vi "CRYCal Perceptual Rub&buzz HarmonicTrack.vi"(6 "Fs":dbl=44100.0, 8 "TSR params":T2={"FSamp"=44100.0, "FStart"=20.0, "FStop"=20000.0, "NOffset"=0.0, "MStop"=132741.0, "MStart"=441.0, "NHarm"=19152.386651933408, "Tsamp"=2.2675736961451248e-05, "Amplit"=1.0, "Sweep Time"=1.0} {"Sweep Time" format="%.2f"; "Amplit" format="%.2f"; "FStop" format="%.2f"; "FStart" format="%.2f"; "FSamp" format="%.2f"; "Tsamp" format="%.2f"; "NHarm" format="%.2f"; "MStart" format="%.2f"; "MStop" format="%.2f"; "NOffset" format="%.2f"}, 9 "Harmonic Infor":T1={"Cycles"=[200.0, 190.0, 180.0, 170.0, 160.0, 150.0, 140.0, 132.0, 125.0, 118.0, 112.0, 106.0, 100.0, 95.0, 90.0, 85.0, 80.0, 75.0, 71.0, 67.0, 63.0, 60.0, 56.0, 53.0, 50.0, 48.0, 45.0, 43.0, 40.0, 38.0, 36.0, 34.0, 32.0, 30.0, 28.0, 27.0, 25.0, 24.0, 23.0, 22.0, 20.0, 19.0, 18.0, 17.0, 16.0, 15.0, 14.0, 14.0, 13.0, 12.0, 12.0, 11.0, 10.0, 10.0, 9.0, 9.0, 8.0, 8.0, 8.0, 7.0, 7.0, 6.0, 6.0, 6.0, 6.0, 6.0, 6.0, 6.0, 6.0, 6.0, 6.0, 6.0, 6.0, 6.0, 8.0, 8.0, 8.0, 8.0, 8.0, 8.0, 8.0, 8.0], "Frequency"=[20000.0, 19000.0, 18000.0, 17000.0, 16000.0, 15000.0, 14000.0, 13199.999809265137, 12500.0, 11800.000190734863, 11199.999809265137, 10600.000381469727, 10000.0, 9500.0, 9000.0, 8500.0, 8000.0, 7500.0, 7099.999904632568, 6699.999809265137, 6300.000190734863, 6000.0, 5599.999904632568, 5300.000190734863, 5000.0, 4750.0, 4500.0, 4250.0, 4000.0, 3750.0, 3549.999952316284, 3349.9999046325684, 3150.0000953674316, 3000.0, 2799.999952316284, 2650.0000953674316, 2500.0, 2359.999895095825, 2240.000009536743, 2119.999885559082, 2000.0, 1900.0, 1800.0, 1700.0, 1600.0, 1500.0, 1400.0, 1319.9999809265137, 1250.0, 1180.0000190734863, 1119.9999809265137, 1060.0000381469727, 1000.0, 950.0, 900.0, 850.0, 800.0, 750.0, 709.9999904632568, 669.9999809265137, 630.0000190734863, 600.0, 559.9999904632568, 530.0000190734863, 500.0, 475.0, 450.0, 425.0, 400.0, 375.0, 354.9999952316284, 334.99999046325684, 315.00000953674316, 300.0, 250.0, 200.0, 160.0, 125.0, 100.0, 80.0, 63.00000190734863, 50.0], "Amplitude"=[0.5, 0.5, 0.5, 0.5, 0.5, 0.5, 0.5, 0.5, 0.5, 0.5, 0.5, 0.5, 0.5, 0.5, 0.5, 0.5, 0.5, 0.5, 0.5, 0.5, 0.5, 0.5, 0.5, 0.5, 0.5, 0.5, 0.5, 0.5, 0.5, 0.5, 0.5, 0.5, 0.5, 0.5, 0.5, 0.5, 0.5, 0.5, 0.5, 0.5, 0.5, 0.5, 0.5, 0.5, 0.5, 0.5, 0.5, 0.5, 0.5, 0.5, 0.5, 0.5, 0.5, 0.5, 0.5, 0.5, 0.5, 0.5, 0.5, 0.5, 0.5, 0.5, 0.5, 0.5, 0.5, 0.5, 0.5, 0.5, 0.5, 0.5, 0.5, 0.5, 0.5, 0.5, 0.5, 0.5, 0.5, 0.5, 0.5, 0.5, 0.5, 0.5], "samples"=[441, 441, 441, 441, 441, 441, 441, 441, 441, 441, 441, 441, 441, 441, 441, 441, 441, 441, 441, 441, 441, 441, 441, 441, 441, 446, 441, 446, 441, 447, 447, 447, 448, 441, 441, 450, 441, 448, 453, 458, 441, 441, 441, 441, 441, 441, 441, 467, 459, 448, 473, 458, 441, 464, 441, 467, 441, 470, 497, 461, 490, 441, 472, 499, 530, 557, 588, 622, 662, 705, 746, 790, 840, 882, 1411, 1764, 2205, 2823, 3528, 4410, 5600, 7055], "Fs"=44100.0, "window"=7, "discard cycles"=1.0} {"discard cycles" min=1.0}, 10 "Response":dbl[](array[numeric]) format="%.2f", 11 "Stimulus":dbl[](array[numeric])=array[132785 elements] format="%.2f") -> (2 "EHS + NL":dbl[](array[numeric]), 3 "Frequency":dbl[](array[numeric]))   [LabVIEW 2013]
panel:
  out "NL Loudness":cluster{"Fc":dbl[], dbl[]}(graph)
  out "EHS Phon":cluster{"Fc":dbl[], dbl[]}(graph)
  out "EHS + NL PHON":cluster{"Fc":dbl[], dbl[]}(graph)
  out "NL Loudness":cluster{"Fc":dbl[], "y out":dbl[]}[](graph)
  out "EHS + NL SPL":cluster{"Fc":dbl[], dbl[]}(graph)
  out "Response Wave":waveform(dbl)(graph)
  out "Stimulus Wave":waveform(dbl)(graph)
  out "EHS":cluster{"Fc":dbl[], dbl[]}(graph)
  out "Hz":dbl
  out "Stimulus dBSPL":cluster{"Fc":dbl[], dbl[]}(graph)
  out "Response dBSPL":cluster{"Fc":dbl[], dbl[]}(graph)
  out "Adapt":cluster{"Freq":dbl[], "EpR":dbl[]}[](graph)
  out "Stimulus EWeight dBSPL":cluster{"Freq":dbl[], "EpR":dbl[]}[](graph)
  out "Response EWeight dBSPL":cluster{"Freq":dbl[], "EpR":dbl[]}[](graph)
  out "Elapsed Time":dbl format="%#_6p"
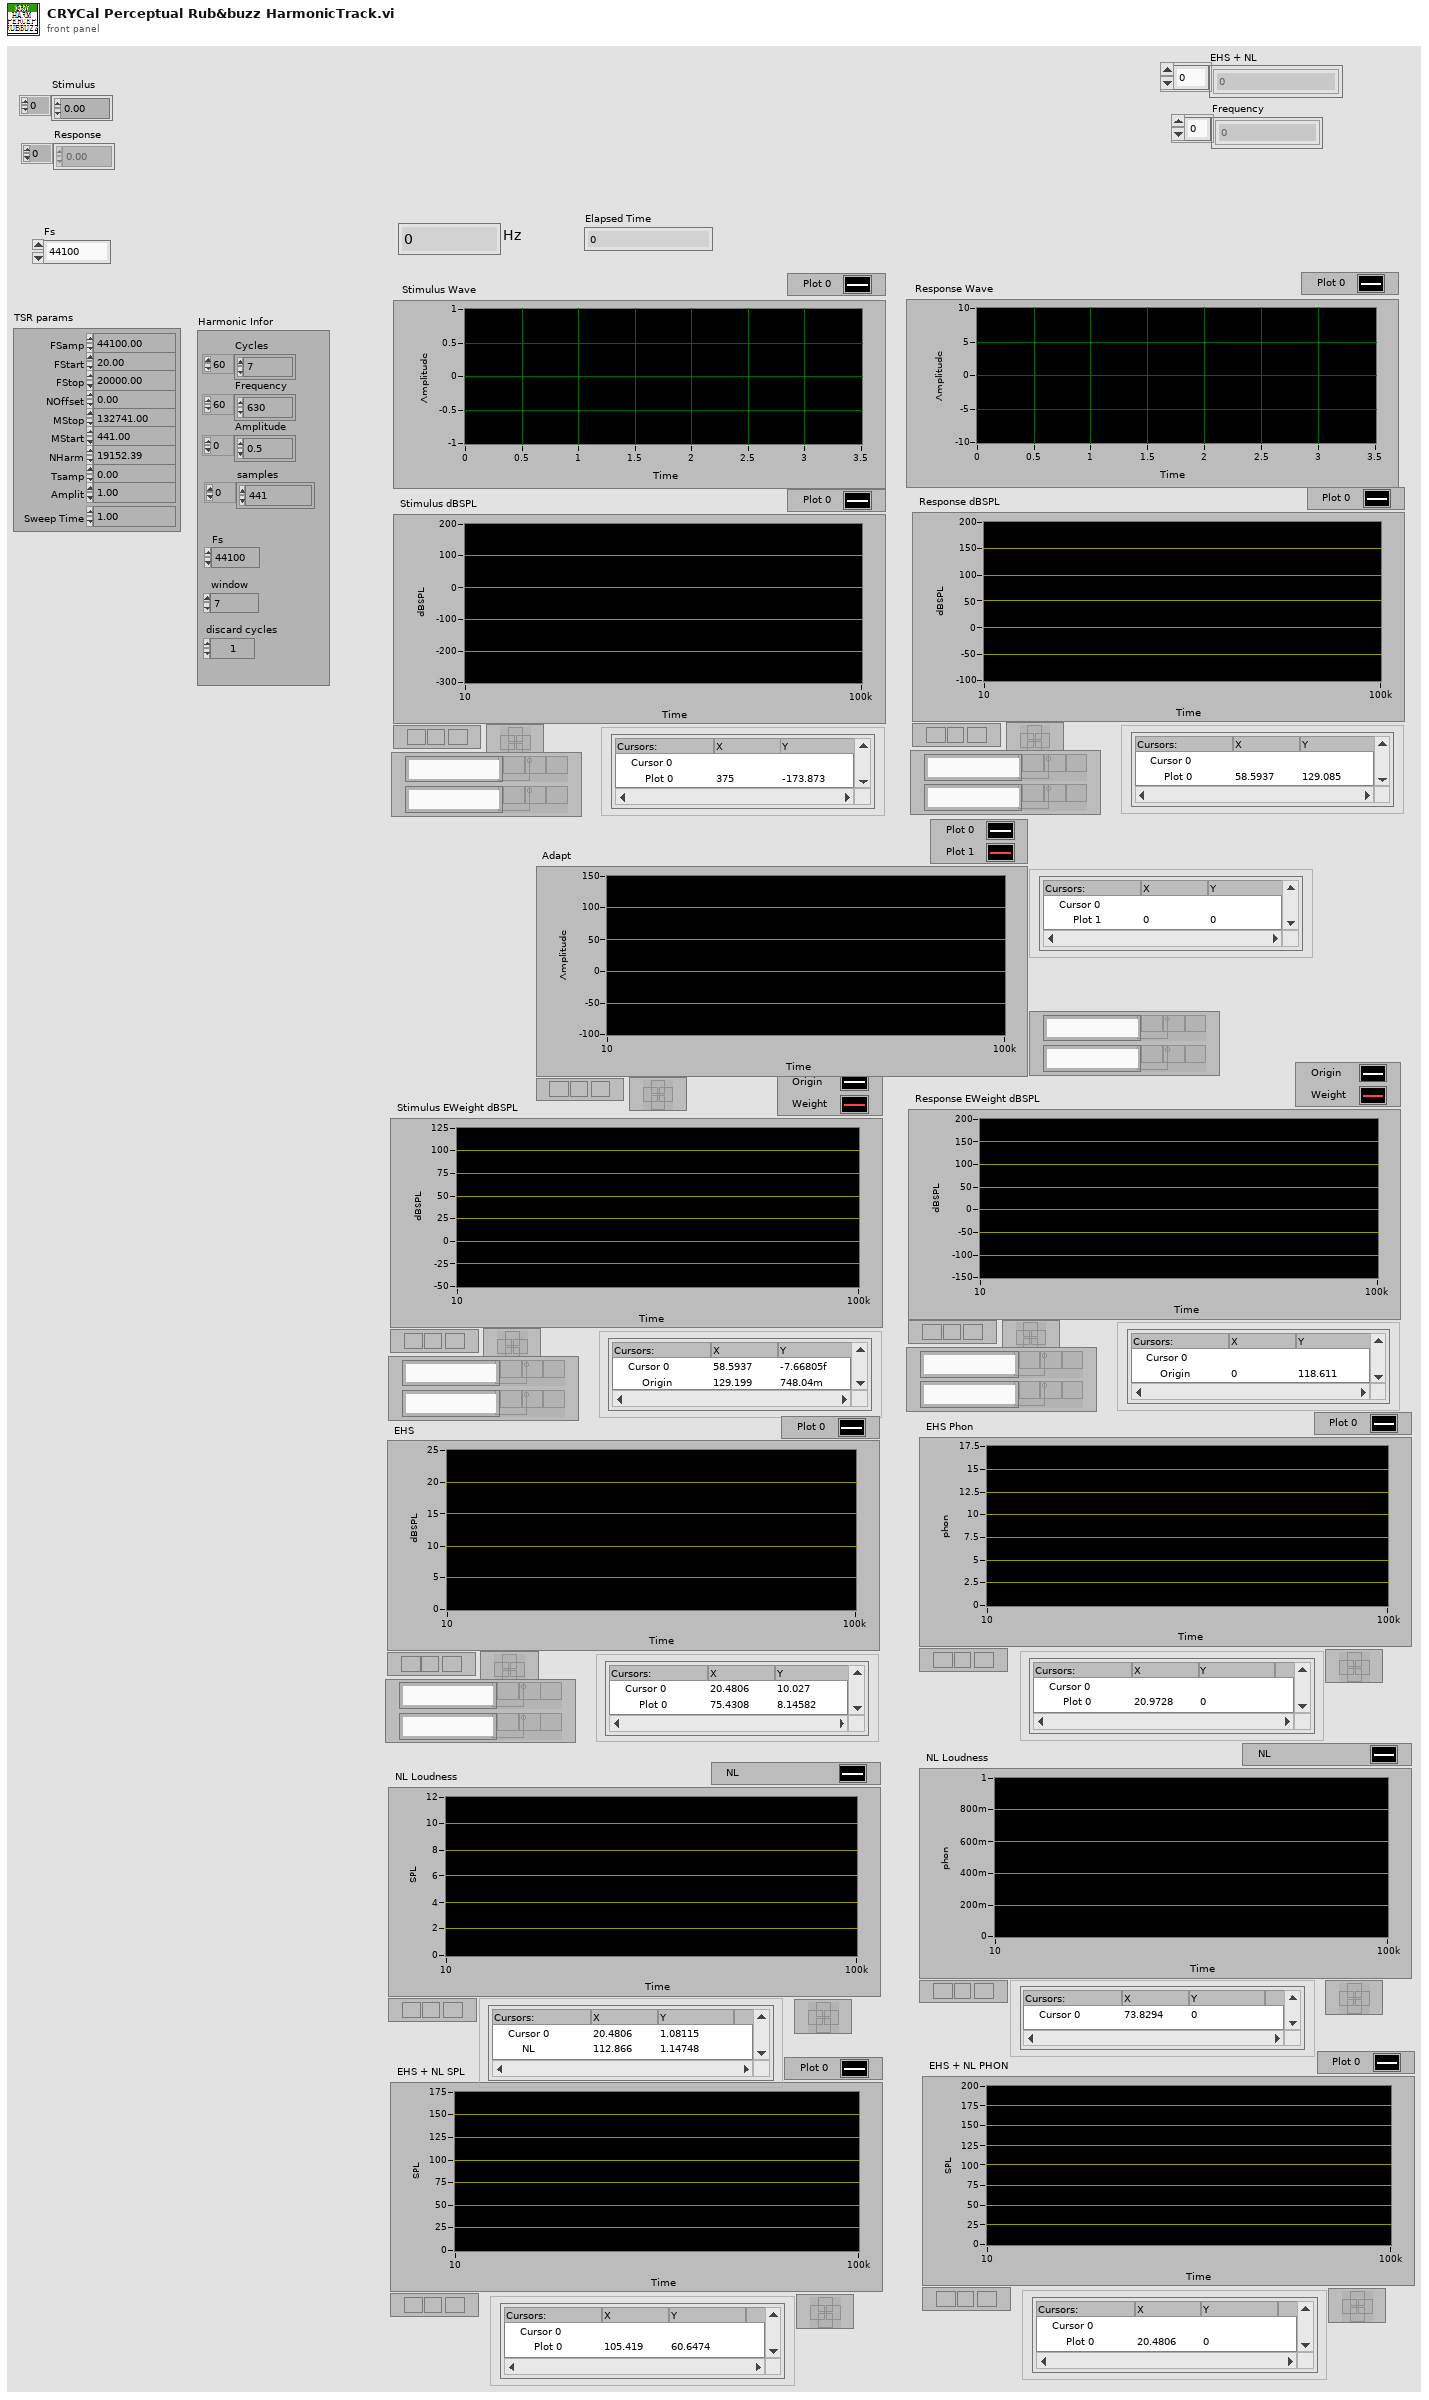
[diagram p1: front panel]
types:
  T1 = cluster{"Cycles":dbl[], "Frequency":dbl[], "Amplitude":dbl[], "samples":i32[], "Fs":dbl, "window":u16, "discard cycles":dbl}
  T2 = cluster{"FSamp":dbl, "FStart":dbl, "FStop":dbl, "NOffset":dbl, "MStop":dbl, "MStart":dbl, "NHarm":dbl, "Tsamp":dbl, "Amplit":dbl, "Sweep Time":dbl}
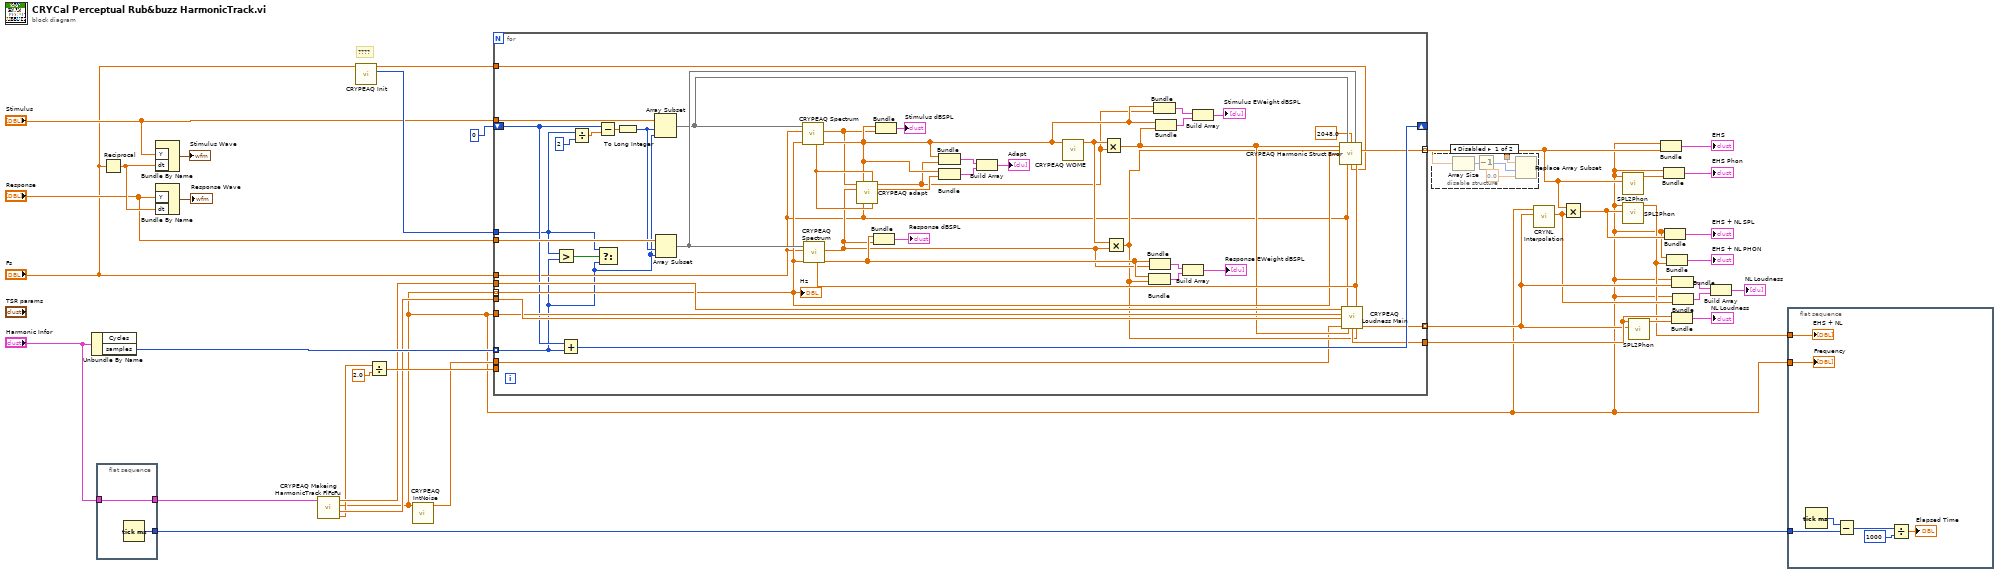
[diagram p0: block diagram]
diagram:
  # "????"
  n1 = Unbundle By Name("Harmonic Infor") -> ("samples"=w7:i32[])  [unwired: 1 out]
  n2 = flat-sequence {
    tunnel: [w38] -> w36
    tunnel: "Harmonic Infor" -> [w37]
    tunnel: [w37] -> w34
    frame #0 {
      n3 = Tick Count (ms)() -> (millisecond timer value=w38:u32)
    }
  }
  n4 = Reciprocal(x="Fs") -> (1/x=w20:dbl)
  n5 = Bundle By Name("Y"="Stimulus", "dt"=w20) -> (→"Stimulus Wave":waveform(dbl))  [unwired: 1 in]
  n6 = Bundle By Name("Y"="Response", "dt"=w20) -> (→"Response Wave":waveform(dbl))  [unwired: 1 in]
  n7 = call "CRYPEAQ Makeing HarmonicTrack FlFcFu.vi"("Harmonic Infor"=w34) -> ("Max Frequency"=w4:dbl, "Fu"=w5:dbl[], "Fc"=w2:dbl[], "Fl"=w6:dbl[])  [unwired: 6 in]
  n8 = call "CRYPEAQ Init.vi"("Fs"="Fs") -> ("Block Size"=w15:i32, "Hanning Window"=w16:dbl[])  [unwired: 9 in]
  n9 = Divide(x=w4, y=2.0) -> (x/y=w30:dbl)
  n10 = call "CRYPEAQ IntNoise.vi"("fc"=w2) -> ("EIN"=w17:dbl[])  [unwired: 10 in]
  n11 = for {
    tunnel: "Stimulus" -> [w68]
    tunnel: "Response" -> [w67]
    tunnel: "Fs" -> [w40]
    shift-right: [w84] -> _
    shift-left: 0 -> [w50]
    tunnel: w7 -> [w39] mode=indexing
    tunnel: w2 -> [w59] mode=indexing
    tunnel: w6 -> [w83]
    tunnel: w5 -> [w77]
    tunnel: w30 -> [_]
    tunnel: w2 -> [w63]
    tunnel: [w70] -> w10 mode=indexing
    tunnel: [w48] -> w21 mode=indexing
    tunnel: [w56] -> w25
    tunnel: w17 -> [w47]
    tunnel: w16 -> [w43]
    tunnel: w15 -> [w41]
    n12 = Greater?(x=w41, y=w39) -> (0:w69:bool)
    n13 = Add(x=w50, y=w39) -> (x+y=w84:i32)
    n14 = Divide(x=w41, y=2) -> (x/y=w45:dbl)
    n15 = Subtract(x=w50, y=w45) -> (x-y=w49:dbl)
    n16 = Select(t=w41, s=w69, f=w39) -> ()  [unwired: 1 out]
    n17 = To Long Integer(number=w49) -> (32bit integer=w44:i32)
    n18 = Array Subset(array=w68, index=w44, length=w39) -> (w57:dbl[])
    n19 = Array Subset(array=w67, index=w44, length=w39) -> (w62:dbl[])
    n20 = call "CRYPEAQ Spectrum.vi"("Freq"=w59, "Fs"=w40, "X"=w57) -> ("Freq"=w58:dbl[], "dBSPL Spectrum"=w55:dbl[], "FFT Size"=w66:dbl)  [unwired: 5 in, 1 out]
    n21 = call "CRYPEAQ Spectrum.vi"("Freq"=w59, "Fs"=w40, "X"=w62) -> ("Freq"=w65:dbl[], "dBSPL Spectrum"=w53:dbl[], "FFT Size"=w64:dbl)  [unwired: 5 in, 1 out]
    n22 = call "CRYPEAQ adapt.vi"("EhsR"=w55, "fc"=w58, "Nc"=w66, "EhsT"=w53, "Fs"=w40, "NF"=w66) -> ("EpR"=w54:dbl[], "EpT"=w60:dbl[])  [unwired: 8 in]
    n23 = Bundle("Freq"=w65, "dBSPL Spectrum"=w53) -> (→"Response dBSPL":cluster{"Freq":dbl[], "dBSPL Spectrum":dbl[]})  [unwired: 1 in]
    n24 = Bundle("Freq"=w58, "dBSPL Spectrum"=w55) -> (→"Stimulus dBSPL":cluster{"Freq":dbl[], "dBSPL Spectrum":dbl[]})  [unwired: 1 in]
    n25 = Bundle("Freq"=w58, "EpR"=w54) -> (w80:cluster{"Freq":dbl[], "EpR":dbl[]})  [unwired: 1 in]
    n26 = Bundle("Freq"=w58, "EpT"=w60) -> (w79:cluster{"Freq":dbl[], "EpT":dbl[]})  [unwired: 1 in]
    n27 = Build Array(w80, w79) -> (→"Adapt":cluster{"Freq":dbl[], "EpT":dbl[]}[])
    n28 = call "CRYPEAQ WOME.vi"("f"=w58) -> ("W2"=w61:dbl[])  [unwired: 10 in]
    n29 = Multiply(x=w61, y=w54) -> (x*y=w52:dbl[])
    n30 = Multiply(x=w61, y=w53) -> (x*y=w51:dbl[])
    n31 = Bundle("Freq"=w65, w51) -> (w73:cluster{"Freq":dbl[], dbl[]})  [unwired: 1 in]
    n32 = Bundle("Freq"=w65, "dBSPL Spectrum"=w53) -> (w72:cluster{"Freq":dbl[], "dBSPL Spectrum":dbl[]})  [unwired: 1 in]
    n33 = Bundle("Freq"=w58, "EpR"=w54) -> (w76:cluster{"Freq":dbl[], "EpR":dbl[]})  [unwired: 1 in]
    n34 = Bundle("Freq"=w58, w52) -> (w75:cluster{"Freq":dbl[], dbl[]})  [unwired: 1 in]
    n35 = Build Array(w72, w73) -> (→"Response EWeight dBSPL":cluster{"Freq":dbl[], "dBSPL Spectrum":dbl[]}[])
    n36 = Build Array(w76, w75) -> (→"Stimulus EWeight dBSPL":cluster{"Freq":dbl[], "EpR":dbl[]}[])
    n37 = call "CRYPEAQ Harmonic Struct Error.vi"("Level Adaptation -> EarWeighted Stimulus"=w52, "Stimulus"=w57, "Correlation Point Number"=2048.0, "Response"=w62, "EarWeighted Response"=w51, "Fc Hz"=w59, "Fs"=w40, "Hanning Window"=w43, "NF"=w64) -> ("EHS"=w70:dbl)  [unwired: 6 in]
    n38 = call "CRYPEAQ Loudness Main.vi"("Fl"=w83, "Fs"=w40, "NF"=w64, "Fc"=w63, "Fu"=w77, "Internal Noise"=w47, "X2R"=w52, "X2T"=w51) -> ("fc"=w56:dbl[], "NL"=w48:dbl)  [unwired: 4 in, 2 out]
    "Hz" <- w59
  }
  n39 = disable-structure shown="Disabled" {
    disable-tunnel: w10 -> [w85 _]
    frame Disabled {
      n40 = Array Size(array=w85) -> (size(s)=w88:i32)
      n41 = Decrement(x=w88) -> (x-1=w87:i32)
      n42 = Replace Array Subset(array=w85, new element=0.0 ("new element/subarray"), index=w87) -> ()  [unwired: 1 out]
    }
    frame Enabled {
    }
  }
  n43 = call "CRYNL Interpolation.vi"("y in"=w21, "x in"=w2) -> ("y out"=w12:dbl[])  [unwired: 9 in]
  n44 = Multiply(x=w10, y=w12) -> (x*y=w22:dbl[])
  n45 = call "SPL2Phon.vi"("SPL in"=w10, "Frequency in"=w2) -> ("Phon out"=w24:dbl[])  [unwired: 9 in]
  n46 = call "SPL2Phon.vi"("SPL in"=w22, "Frequency in"=w2) -> ("Phon out"=w3:dbl[])  [unwired: 9 in]
  n47 = call "SPL2Phon.vi"("SPL in"=w21, "Frequency in"=w25) -> ("Phon out"=w23:dbl[])  [unwired: 9 in]
  n48 = Bundle("Fc"=w2, w10) -> (→"EHS":cluster{"Fc":dbl[], dbl[]})  [unwired: 1 in]
  n49 = Bundle("Fc"=w2, "Phon out"=w24) -> (→"EHS Phon":cluster{"Fc":dbl[], "Phon out":dbl[]})  [unwired: 1 in]
  n50 = Bundle("Fc"=w2, w22) -> (→"EHS + NL SPL":cluster{"Fc":dbl[], dbl[]})  [unwired: 1 in]
  n51 = Bundle("Fc"=w2, "Phon out"=w3) -> (→"EHS + NL PHON":cluster{"Fc":dbl[], "Phon out":dbl[]})  [unwired: 1 in]
  n52 = Bundle("fc"=w25, "Phon out"=w23) -> (→"NL Loudness":cluster{"fc":dbl[], "Phon out":dbl[]})  [unwired: 1 in]
  n53 = Bundle("Fc"=w2, w21) -> (w14:cluster{"Fc":dbl[], dbl[]})  [unwired: 1 in]
  n54 = Bundle("Fc"=w2, "y out"=w12) -> (w13:cluster{"Fc":dbl[], "y out":dbl[]})  [unwired: 1 in]
  n55 = Build Array(w14, w13) -> (→"NL Loudness":cluster{"Fc":dbl[], "y out":dbl[]}[])
  n56 = flat-sequence {
    tunnel: w36 -> [w94]
    tunnel: w2 -> [w90]
    tunnel: w3 -> [w89]
    frame #0 {
      n57 = Tick Count (ms)() -> (millisecond timer value=w95:u32)
      n58 = Subtract(x=w95, y=w94) -> (x-y=w93:u32)
      n59 = Divide(x=w93, y=u32 1000) -> (x/y=→"Elapsed Time":dbl)
      "Frequency" <- w90
      "EHS + NL" <- w89
    }
  }
